vi "libssh2_knownhost_writefile.vi"(8 "error in (no error)":errorcluster, 9 "type":i32, 10 "filename":string, 11 "known hosts":T1) -> (0 "error out":errorcluster, 3 "return value":i32)   [LabVIEW 2013, in "libssh2.lvlib"]
doc: "Writes all known hosts to the specified file using the specified file format."
uses:
  libssh2.lvlib
  Known Hosts Refnum.ctl
  libssh2.dll
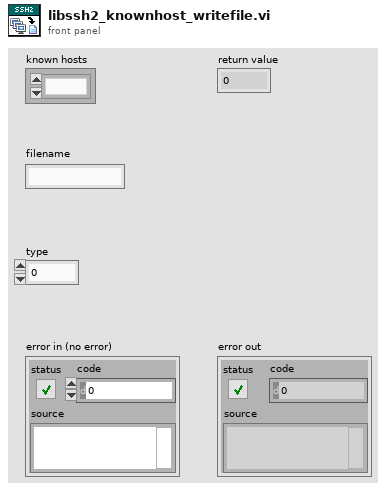
[diagram p1: front panel]
types:
  T1 = typedef "libssh2.lvlib/Known Hosts Refnum.ctl" = refnum<k1>
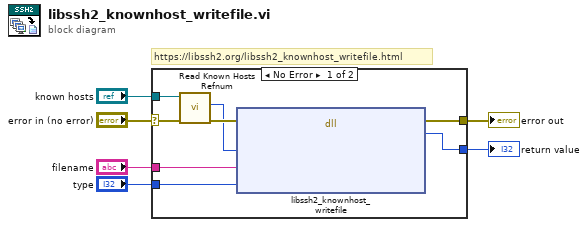
[diagram p0: block diagram]
diagram:
  # "https://libssh2.org/libssh2_knownhost_writefile.html"
  n1 = case shown="No Error" "error in (no error)" {
    selector: "error in (no error)" -> [w7 w15]
    tunnel: [w14 _] -> w6
    tunnel: [w13 w15] -> w5
    tunnel: "filename" -> [w12 _]
    tunnel: "type" -> [w11 _]
    tunnel: "known hosts" -> [w9 _]
    frame No Error {
      n2 = call "Read Known Hosts Refnum.vi"("error in (no error)"=w7, "known hosts"=w9) -> ("error out"=w10:errorcluster, "LIBSSH2_KNOWNHOSTS*"=w8:u64)  [unwired: 8 in]
      n3 = dll-call lib="C:/Users/pasca/source/repos/libssh2-labview/libssh2**.*" fn="libssh2_knownhost_writefile"(error in=w10, "hosts"=w8, "filename"=w12, "type"=w11) -> (error out=w13:errorcluster, "return value"=w14:i32)  [unwired: 5 in, 1 out]
    }
    frame Error {
    }
  }
  "return value" <- w6
  "error out" <- w5
